vi "add_image_to_file.vi"(0 "Cluster d'image":cluster{"Heure":string, "Array":i32[][]}, 1 "Chemin du fichier de guidage":path) -> ()   [LabVIEW 2011]
panel:
  out "Array d'images":cluster{"Heure":string, "Array":i32[][]}[](array[cluster])
  # "Exécution en < 20ms pour 48 images !!!\nsoit 4h avec enregistrement toutes les 5 mins"
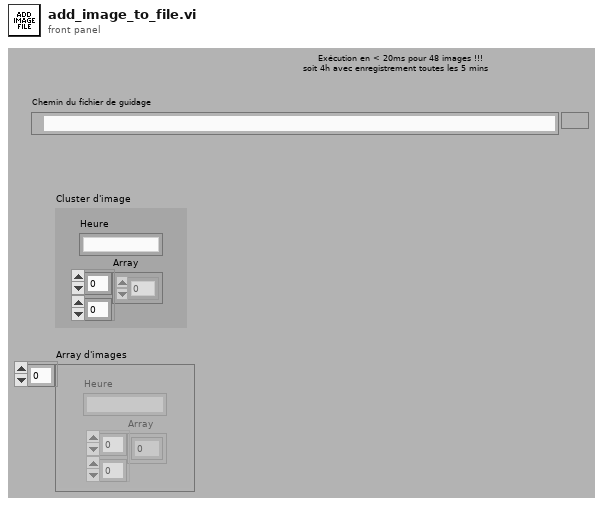
[diagram p1: front panel]
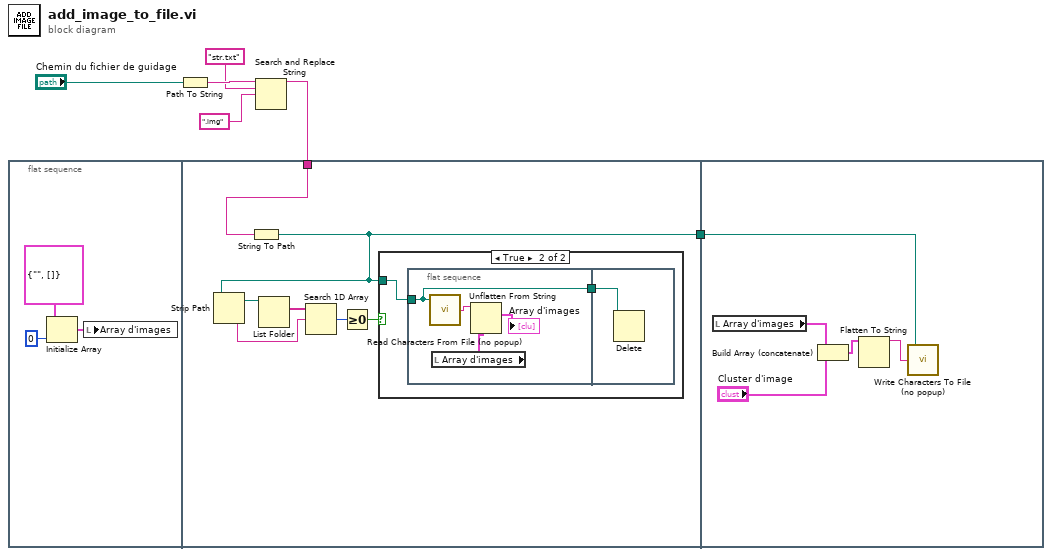
[diagram p0: block diagram]
diagram:
  n1 = flat-sequence {
    tunnel: [w11] -> w6
    tunnel: w1 -> [w10]
    tunnel: w6 -> [w25]
    frame #0 {
      n2 = Initialize Array(cluster{string, i32[][]} {"", []}, 0 ("dimension size")) -> (w9:cluster{string, i32[][]}[])
      n3 = local write "Array d'images"(w9) -> ()
    }
    frame #1 {
      n4 = String To Path(string=w10) -> (path=w11:path)
      n5 = Strip Path(path=w11) -> (stripped path=w16:path, name=w15:string)
      n6 = List Folder(path=w16) -> (filenames=w14:string[])  [unwired: 3 in, 3 out]
      n7 = Search 1D Array(1D array=w14, element=w15) -> (index of element=w13:i32)  [unwired: 1 in]
      n8 = Greater Or Equal To 0?(x=w13) -> (x >= 0?=w12:bool)
      n9 = case shown="True" w12 {
        tunnel: w11 -> [_ w18]
        frame False {
        }
        frame True {
          n10 = flat-sequence {
            tunnel: w18 -> [w19]
            tunnel: [w19] -> w17
            tunnel: w17 -> [w23]
            frame #0 {
              n11 = call "Read Characters From File (no popup).vi"("file path (dialog if empty)"=w19) -> ("character string"=w22:string)  [unwired: 5 in, 3 out]
              n12 = local read "Array d'images"() -> (w20:cluster{"Heure":string, "Array":i32[][]}[])
              n13 = Unflatten From String(type=w20, binary string=w22) -> (value=→"Array d'images":cluster{"Heure":string, "Array":i32[][]}[])  [unwired: 3 in, 2 out]
            }
            frame #1 {
              n14 = Delete(path (use dialog)=w23) -> ()  [unwired: 4 in, 3 out]
            }
          }
        }
      }
    }
    frame #2 {
      n15 = local read "Array d'images"() -> (w28:cluster{"Heure":string, "Array":i32[][]}[])
      n16 = Build Array (concatenate)(w28, "Cluster d'image") -> (w26:cluster{"Heure":string, "Array":i32[][]}[])
      n17 = Flatten To String(anything=w26) -> (data string=w24:string)  [unwired: 3 in, 2 out]
      n18 = call "Write Characters To File (no popup).vi"("character string"=w24, "file path (dialog if empty)"=w25) -> ()  [unwired: 3 in, 1 out]
    }
  }
  n19 = Path To String(path="Chemin du fichier de guidage") -> (string=w4:string)
  n20 = Search and Replace String(input string=w4, search string="str.txt", replace string=".img" ("search string")) -> (result string=w1:string)  [unwired: 5 in, 3 out]
